vi "orangeLocation.vi"() -> (0 "Orange_Data":dbl[](array[numeric]), 1 "orange_stop":bool)   [LabVIEW 2017]
panel:
  out "Numeric":i32
  out "size(s)":i32
  # "center x"
  # "center y"
  # "left"
  # "up"
  # "right"
  # "bot"
  # "width"
  # "height"
  # "tayang"
  # "area"
  # "convex hull area"
  # "img area"
  # "%area/img area"
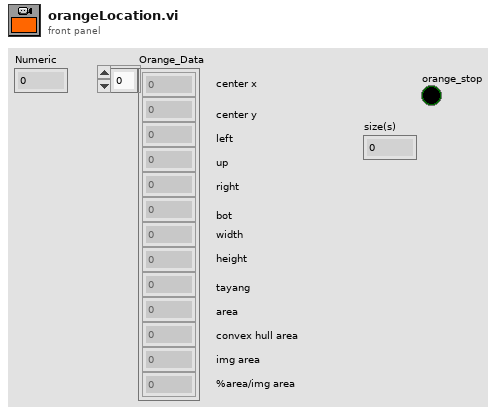
[diagram p1: front panel]
types:
  T1 = typedef "IMAQ Image.ctl" = refnum<image>
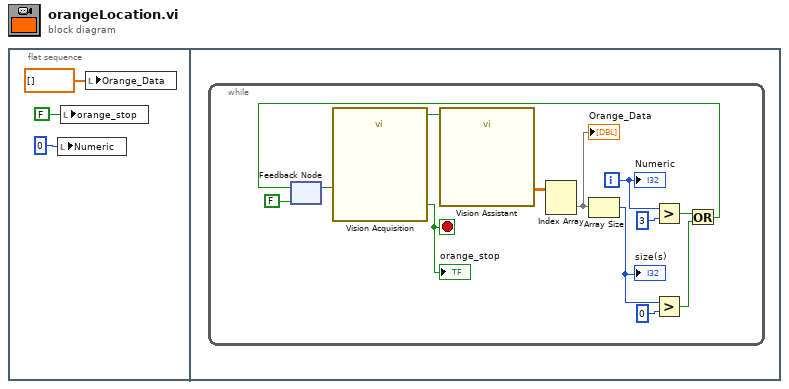
[diagram p0: block diagram]
diagram:
  n1 = flat-sequence {
    frame #0 {
      n2 = local write "Numeric"(0 ("Numeric")) -> ()
      n3 = local write "orange_stop"(FALSE ("orange_stop")) -> ()
      n4 = local write "Orange_Data"(dbl[] [] ("Orange_Data")) -> ()
    }
    frame #1 {
      n5 = while {
        i -> [w10]
        stop <- w5 stop-if-true
        n6 = feedback #1(FALSE) -> (w6:bool)
        n7 = call "Vision Acquisition"("Stop (F)"=w6) -> ("Image Out"=w16:T1, "Stopped"=w5:bool)  [unwired: 24 in, 1 out]
        "orange_stop" <- w5
        n8 = call "Vision Assistant"("Image In"=w16) -> ("Particle Measurements (Pixels) (Particle Analysis 1)"=w15:dbl[][])  [unwired: 23 in, 3 out]
        n9 = Index Array(array=w15) -> (element=w12:dbl[])  [unwired: 2 in]
        "Orange_Data" <- w12
        n10 = Array Size(array=w12) -> (size(s)=w14:i32)
        "size(s)" <- w14
        n11 = Greater?(x=w10, y=3) -> (0:w8:bool)
        n12 = Greater?(x=w14, y=0) -> (0:w11:bool)
        n13 = Or(x=w8, y=w11) -> (x .or. y?=w7:bool)
        n14 = feedback-in #1(w7) -> ()
        "Numeric" <- w10
      }
    }
  }
